vi "write multipart text.vi"(10 "text":string[](array[string]), 11 "websocket client in":refnum<class "websocket client.lvclass">) -> (0 "error out":errorcluster, 3 "websocket client out":refnum<class "websocket client.lvclass">)   [LabVIEW 2016, in "websocket client.lvclass"]
uses:
  websocket client.lvclass
  websocket client.lvclass/websocket client.ctl
  opcode.ctl
  websocket core.lvlib
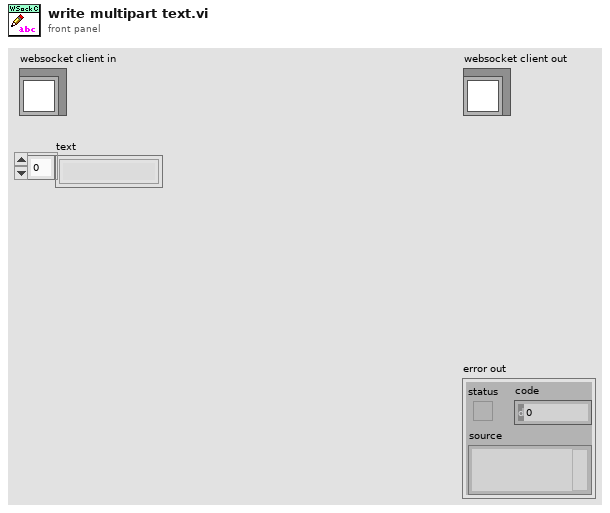
[diagram p1: front panel]
types:
  T1 = typedef "websocket core.lvlib/opcode.ctl" = u8
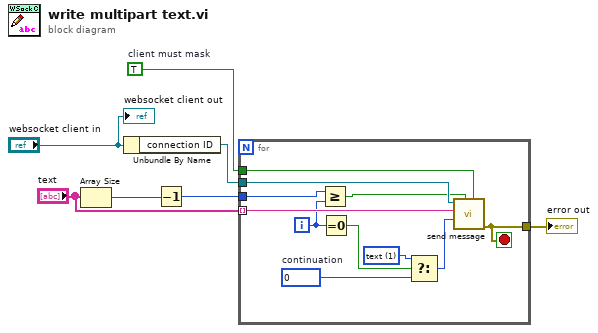
[diagram p0: block diagram]
diagram:
  w4 = TRUE  # client must mask
  n1 = Array Size(array="text") -> (size(s)=w2:i32)
  n2 = Unbundle By Name("websocket client in") -> ("connection ID"=w6:refnum<k5>)
  n3 = Decrement(x=w2) -> (x-1=w1:i32)
  n4 = for {
    tunnel: w6 -> [w18]
    tunnel: [w16] -> w5
    tunnel: w4 -> [w17]
    tunnel: "text" -> [w11] mode=indexing
    tunnel: w1 -> [w10]
    i -> [w9]
    stop <- w16 stop-if-true
    w13 = T1 0 items=["text"=1, "binary"=2, "x3"=3, "x4"=4, "x5"=5, "x6"=6, "x7"=7]  # continuation
    w14 = T1 1 items=["text"=1, "binary"=2, "x3"=3, "x4"=4, "x5"=5, "x6"=6, "x7"=7] ("opcode")
    n5 = Greater Or Equal?(x=w10, y=w9) -> (x >= y?=w8:bool)
    n6 = Equal To 0?(x=w9) -> (x = 0?=w15:bool)
    n7 = Select(t=w14, s=w15, f=w13) -> (s? t:f=w12:T1)
    n8 = call "send message.vi"("mask? (F)"=w17, "final fragment (T)"=w8, "opcode"=w12, "data"=w11, "TCP Network Connection in"=w18) -> ("error out"=w16:errorcluster)  [unwired: 6 in]
  }
  "error out" <- w5
  "websocket client out" <- "websocket client in"
